vi "ANAL_TreeString.vi"(11 "Main Data Array":T2 {"Run Data Cluster"."Temperature B" scale=0.0..100.0; "Run Data Cluster"."Temperature A" scale=0.0..100.0}) -> (2 "Tree Cluster Out":T1, 3 "Main Data Array 2":T2 {"Run Data Cluster"."Temperature B" scale=0.0..100.0; "Run Data Cluster"."Temperature A" scale=0.0..100.0})   [LabVIEW 2021]
uses:
  ANAL_Data.ctl
  XML_Cluster.ctl
  DAT_Cluster.ctl
  ANAL_TREECluster.ctl
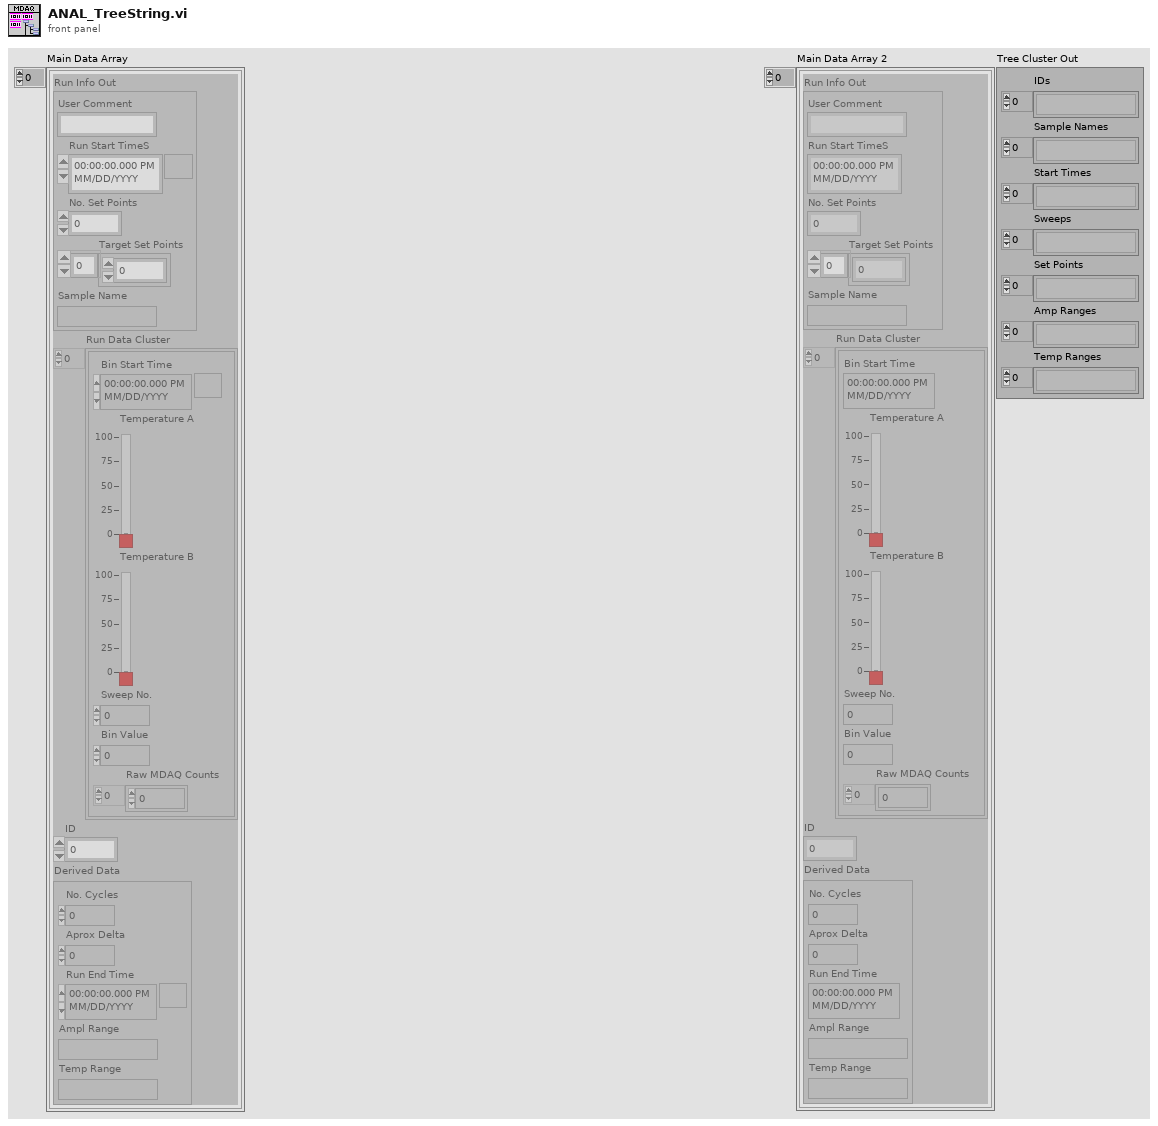
[diagram p1: front panel]
types:
  T1 = typedef "ANAL_TREECluster.ctl" = cluster{"IDs":string[], "Sample Names":string[], "Start Times":string[], "Sweeps":string[], "Set Points":string[], "Amp Ranges":string[], "Temp Ranges":string[]}
  T2 = typedef "ANAL_Data.ctl" = cluster{"Run Info Out":T3, "Run Data Cluster":T4, "ID":u32, "Derived Data":cluster{"No. Cycles":u32, "Aprox Delta":dbl, "Run End Time":timestamp, "Ampl Range":string, "Temp Range":string}}[]
  T3 = typedef "XML_Cluster.ctl" = cluster{"User Comment":string, "Run Start TimeS":timestamp, "No. Set Points":u32, "Target Set Points":i32[], "Sample Name":string}
  T4 = typedef "DAT_Cluster.ctl" = cluster{"Bin Start Time":timestamp, "Temperature A":dbl, "Temperature B":dbl, "Sweep No.":i32, "Bin Value":i32, "Raw MDAQ Counts":i32[]}[]
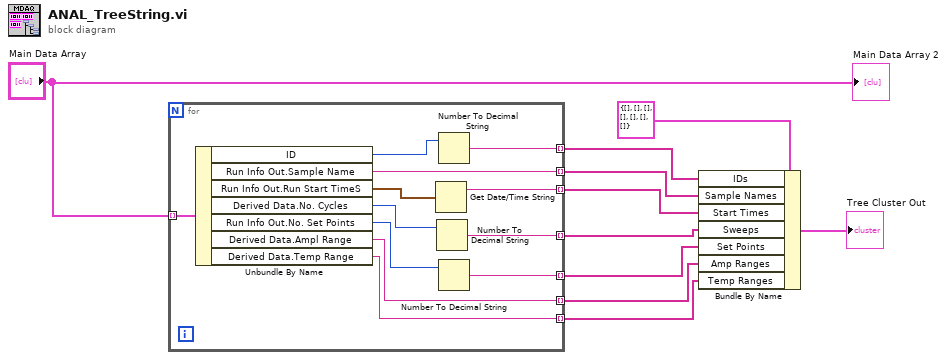
[diagram p0: block diagram]
diagram:
  n1 = for {
    tunnel: "Main Data Array" -> [w22] mode=indexing
    tunnel: [w21] -> w7 mode=indexing
    tunnel: [w19] -> w6 mode=indexing
    tunnel: [w17] -> w5 mode=indexing
    tunnel: [w16] -> w4 mode=indexing
    tunnel: [w14] -> w3 mode=indexing
    tunnel: [w13] -> w2 mode=indexing
    tunnel: [w11] -> w8 mode=indexing
    n2 = Unbundle By Name(w22) -> ("ID"=w12:u32, "Run Info Out.Sample Name"=w21:string, "Run Info Out.Run Start TimeS"=w20:timestamp, "Derived Data.No. Cycles"=w18:u32, "Run Info Out.No. Set Points"=w15:u32, "Derived Data.Ampl Range"=w14:string, "Derived Data.Temp Range"=w13:string)
    n3 = Get Date/Time String(seconds (now)=w20) -> (date string=w19:string)  [unwired: 2 in, 1 out]
    n4 = Number To Decimal String(number=w18) -> (decimal integer string=w17:string)  [unwired: 1 in]
    n5 = Number To Decimal String(number=w12) -> (decimal integer string=w11:string)  [unwired: 1 in]
    n6 = Number To Decimal String(number=w15) -> (decimal integer string=w16:string)  [unwired: 1 in]
  }
  n7 = Bundle By Name(cluster=T1 {"IDs"=[], "Sample Names"=[], "Start Times"=[], "Sweeps"=[], "Set Points"=[], "Amp Ranges"=[], "Temp Ranges"=[]} ("Tree Data Cluster"), "IDs"=w8, "Sample Names"=w7, "Start Times"=w6, "Sweeps"=w5, "Set Points"=w4, "Amp Ranges"=w3, "Temp Ranges"=w2) -> (→"Tree Cluster Out":T1)
  "Main Data Array 2" <- "Main Data Array"
